vi "SetTriggerDirection.vi"(8 "Error In":errorcluster, 10 "Trigger Direction":T1, 11 "Keithley 6485 In":refnum<visa-resource-name>) -> (0 "Error Out":errorcluster, 3 "Keithley 6485 Out":refnum<visa-resource-name>)   [LabVIEW 2012, in "Keithley-6485.lvlib"]
uses:
  Keithley-6485.lvlib
  Controls/TriggerDirection.ctl
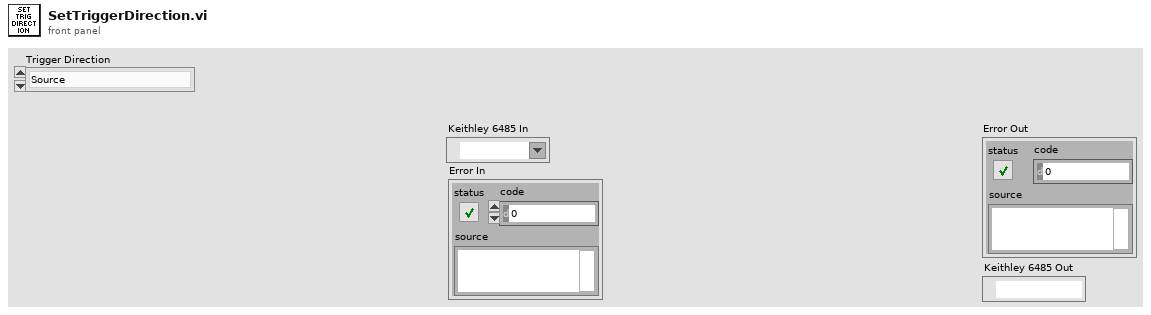
[diagram p1: front panel]
types:
  T1 = typedef "Keithley-6485.lvlib/TriggerDirection.ctl" = enum16{"Source", "Acceptor"}
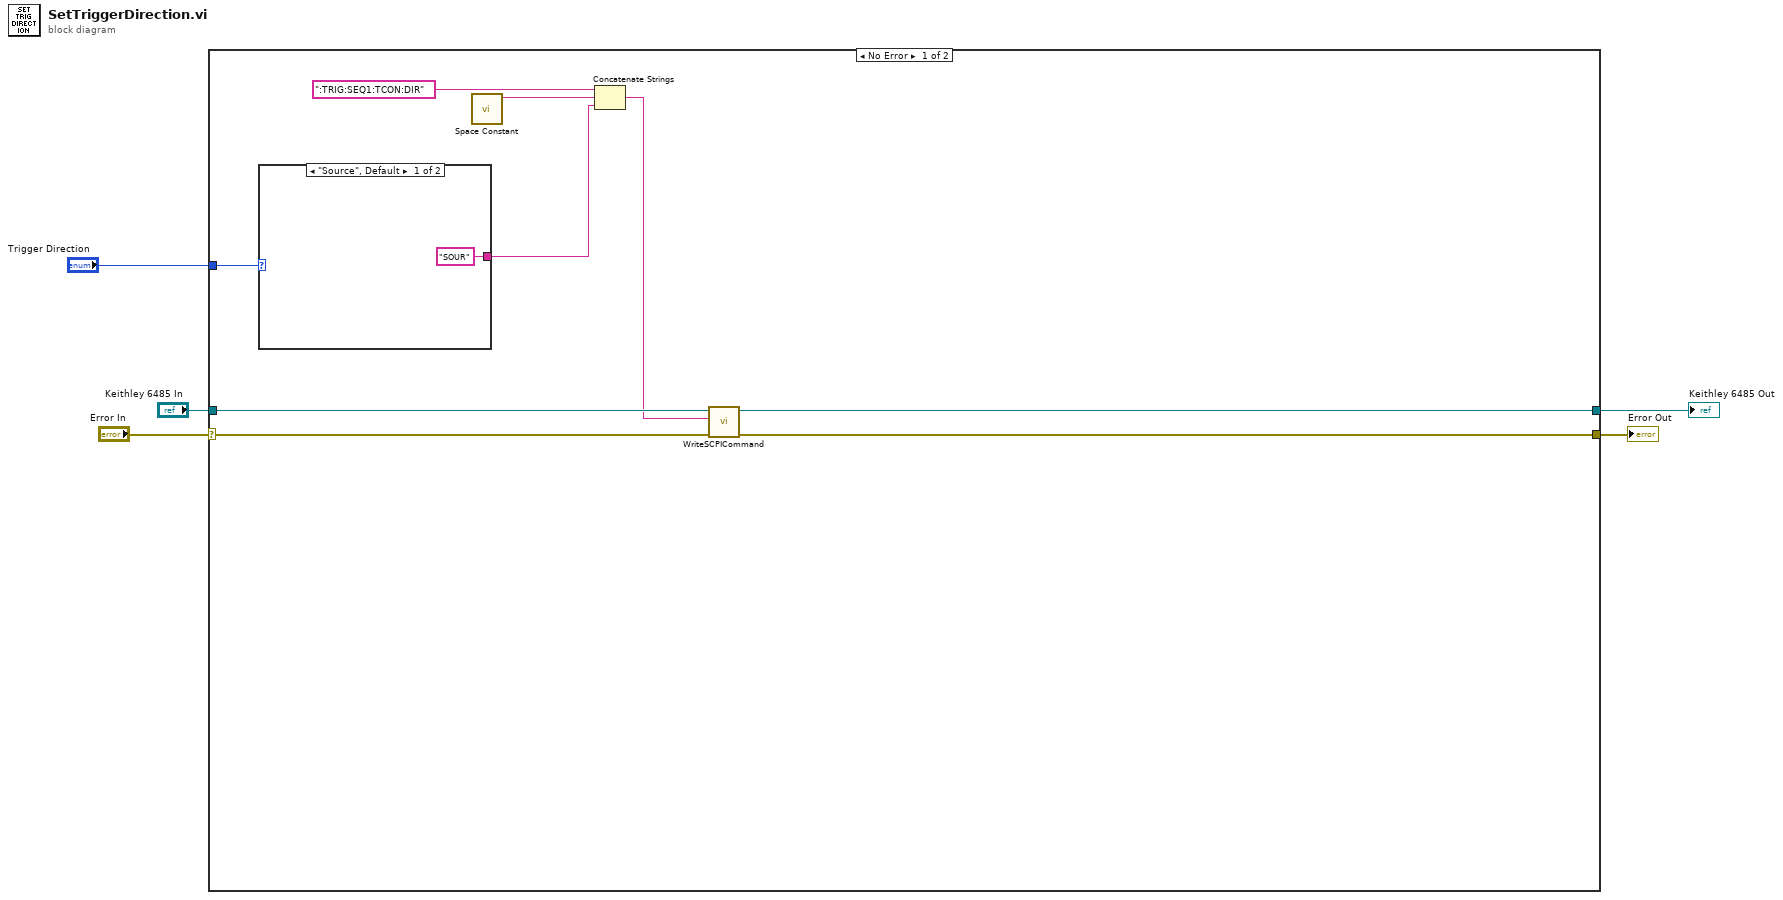
[diagram p0: block diagram]
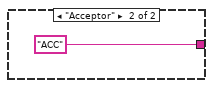
[diagram p2: hidden frame]
diagram:
  n1 = case shown="No Error" "Error In" {
    selector: "Error In" -> [w14 w17]
    tunnel: "Keithley 6485 In" -> [w13 w18]
    tunnel: [w8 w17] -> w3
    tunnel: [w9 w18] -> w2
    tunnel: "Trigger Direction" -> [w6 _]
    frame No Error {
      n2 = case shown="\"Source\", Default" w6 {
        tunnel: ["SOUR" "ACC"] -> w7
        frame "Source", Default {
        }
        frame "Acceptor" {
        }
      }
      n3 = call <vilib>:"Space Constant.vi"() -> ("String"=w11:string)
      n4 = Concatenate Strings(":TRIG:SEQ1:TCON:DIR" ("string"), w11, w7) -> (w10:string)
      n5 = call "WriteSCPICommand.vi"("Error In"=w14, "SCPI Command"=w10, "Keithley 6482 In"=w13) -> ("Error Out"=w8:errorcluster, "Keithley 6482 Out"=w9:refnum<visa-resource-name>)  [unwired: 7 in]
    }
    frame Error {
    }
  }
  "Error Out" <- w3
  "Keithley 6485 Out" <- w2
